vi "getClassName.vi"(8 "error in (no error)":errorcluster, 11 "DataObj in":refnum<class "DataObj.lvclass">) -> (0 "error out":errorcluster, 2 "name":string, 3 "DataObj out":refnum<class "DataObj.lvclass">)   [LabVIEW 2009, in "DataObj.lvclass"]
doc: "Return the name of the class."
uses:
  DataObj.lvclass
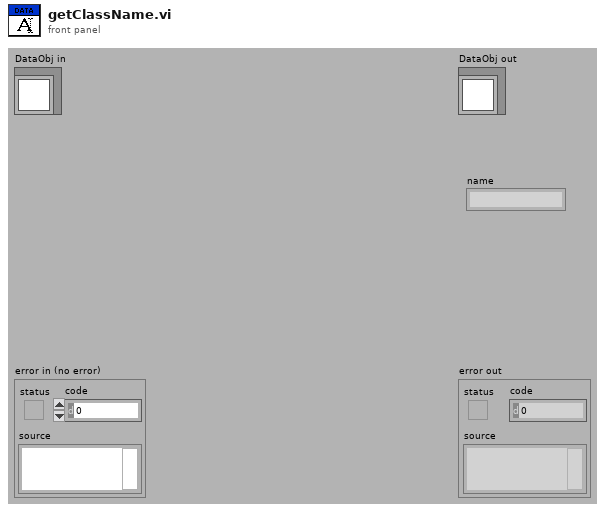
[diagram p1: front panel]
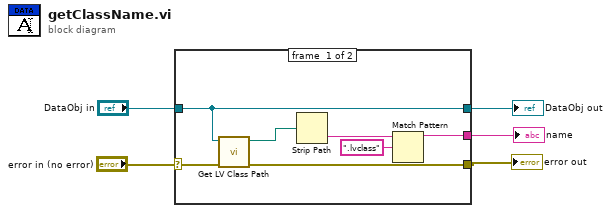
[diagram p0: block diagram]
diagram:
  n1 = case shown="No Error" "error in (no error)" {
    selector: "error in (no error)" -> [w11 w14]
    tunnel: [w7 w14] -> w2
    tunnel: [w12 w13] -> w4
    tunnel: "DataObj in" -> [w12 w13]
    tunnel: [w6 _] -> w1
    frame #0 {
      n2 = call <vilib>:"Get LV Class Path.vi"("error in (no error)"=w11, "object"=w12) -> ("error out"=w7:errorcluster, "class path"=w10:path)  [unwired: 8 in]
      n3 = Strip Path(path=w10) -> (name=w9:string)  [unwired: 1 out]
      n4 = Match Pattern(string=w9, regular expression=".lvclass") -> (before substring=w6:string)  [unwired: 1 in, 3 out]
    }
    frame #1 {
    }
  }
  "error out" <- w2
  "DataObj out" <- w4
  "name" <- w1
